vi "Host - Send Serial CMD (SubVI).vi"(5 "Access Restricted?":bool, 7 "Values":dbl[](array[numeric]), 10 "Camera Controls":T3, 11 "Data Cluster":T4={"VI References"=[], "Addresses"=[], "Pilot"=FALSE, "DO Data"=[], "Access Restricted?"=FALSE, "Pilot Control References"=[], "CoPilot Control References"=[], "cRIO Config"=[], "datalog Q"=refnum, "PS_P"={"AI"=[], "DI"=[], "DO"=[], "Serial"=[], "CPU"={"Total Load"=[], "Interrupt Load"=[], "Total Physical"=0.0, "Free Physical"=0.0, "Primary Disk Capacity"=0.0, "Primary Disk Free"=0.0}, "Stop"=FALSE, "DO Channel"=[]}, "PS_S"={"AI"=[], "DI"=[], "DO"=[], "Serial"=[], "CPU"={"Total Load"=[], "Interrupt Load"=[], "Total Physical"=0.0, "Free Physical"=0.0, "Primary Disk Capacity"=0.0, "Primary Disk Free"=0.0}, "Stop"=FALSE, "DO Channel"=[]}, "IDE_P"={"AI"=[], "DI"=[], "DO"=[], "Serial"=[], "CPU"={"Total Load"=[], "Interrupt Load"=[], "Total Physical"=0.0, "Free Physical"=0.0, "Primary Disk Capacity"=0.0, "Primary Disk Free"=0.0}, "Stop"=FALSE, "DO Channel"=[]}, "IDE_S"={"AI"=[], "DI"=[], "DO"=[], "Serial"=[], "CPU"={"Total Load"=[], "Interrupt Load"=[], "Total Physical"=0.0, "Free Physical"=0.0, "Primary Disk Capacity"=0.0, "Primary Disk Free"=0.0}, "Stop"=FALSE, "DO Channel"=[]}, "PDE_P"={"AI"=[], "DI"=[], "DO"=[], "Serial"=[], "CPU"={"Total Load"=[], "Interrupt Load"=[], "Total Physical"=0.0, "Free Physical"=0.0, "Primary Disk Capacity"=0.0, "Primary Disk Free"=0.0}, "Stop"=FALSE, "DO Channel"=[]}, "PDE_S"={"AI"=[], "DI"=[], "DO"=[], "Serial"=[], "CPU"={"Total Load"=[], "Interrupt Load"=[], "Total Physical"=0.0, "Free Physical"=0.0, "Primary Disk Capacity"=0.0, "Primary Disk Free"=0.0}, "Stop"=FALSE, "DO Channel"=[]}, "GUI References"={"Control Names"=[], "Control References"=[]}, "GUI Data"=[], "TCP - Serial"=[], "TCP-Serial Q"=refnum, "TCP Serial Ref"=[], "Data Sets"=[], "Last Data"=[], "Alarm Data"=[], "DI Data"=[], "Ack Data"=[], "Buzzer Data"=[], "Pilot DO"=[], "Co-Pilot DO"=[], "System Down?"=FALSE, "Log Data"=[], "Update Array"=[], "MCC Data Log"=[], "MCC Data Not"=refnum, "Thruster control"=[refnum, refnum, refnum, refnum, refnum, refnum, refnum, refnum, refnum], "waga notifier out"=refnum, "Wago  log"=[], "Thruster Cont"=[0.0, 0.0, 0.0, 0.0, 0.0, 0.0, 0.0, 0.0, 0.0], "Cam Cont"=[FALSE, FALSE, FALSE, FALSE, FALSE, TRUE], "PDE_P TH Cont"={"COM 10"=0.0, "COM 11"=0.0, "COM 12"=0.0, "COM 13"=0.0}, "PDE_S TH Cont"={"COM 10"=0.0, "COM 11"=0.0, "COM 12"=0.0, "COM 13"=0.0}} {"cRIO Config"."AI"."Interface Data"."Timing"."sample mode" items=["Finite Samples"=10178, "Continuous Samples"=10123, "Hardware Timed Single Point"=12522]; "cRIO Config"."Async"."Interface Data"."Data"."Minor Frame Count" min=5 max=8 step=1}) -> (2 "# elements in queue":i32)   [LabVIEW 2021]
uses:
  Controls/Host - GUI Data Cluster.ctl
  Analog Output/Controls/AO JSON Data Cluster.ctl
  Analog Output/Controls/AO Interface Data Cluster.ctl
  Analog Output/Controls/AO Channel Configuration Cluster.ctl
  Analog Output/Controls/AO Timing Cluster.ctl
  Digital Output/Controls/DIO Configuration cluster.ctl
  Digital Output/Controls/DIO Interface Data.ctl
  Digital Output/SubVIs/Digital Dynamic Cluster.ctl
  Async JSON Cluster.ctl
  Async Interface Data Cluster.ctl
  Async Serial/Controls/Async Serial Configuration Cluster.ctl
  Async Serial/Controls/Async Frame Info Cluster.ctl
  Async Serial/Controls/Async Message Info Cluster.ctl
  Controls/Host Data Cluster.ctl
  Main Engine/Controls/Main Engine CPU Info.ctl
  <userlib>/_OpenG.lib/comparison/comparison.llb/1D DBL Array Changed__ogtk.vi
  Controls/Global Variable.vi
  <userlib>/_OpenG.lib/comparison/comparison.llb/openg_comparison__ogtk.lvlib
panel:
  out "Changed":bool
  in  "Frame Info 2":T1[](array[typedef])=[{"Frame ID"=1, "Message Info"=[{"Message"=[16, 1, 111, 65, 32, 32, 0, 0, 16, 3, 20, 16, 1, 111, 65, 32, 32, 0, 0, 16, 3, 5], "Message Name"="cmd"}]}, {"Frame ID"=1, "Message Info"=[{"Message"=[16, 1, 111, 65, 32, 32, 0, 0, 16, 3, 20, 16, 1, 111, 65, 32, 32, 0, 0, 16, 3, 5], "Message Name"="cmd"}]}, {"Frame ID"=1, "Message Info"=[{"Message"=[16, 1, 111, 65, 32, 32, 0, 0, 16, 3, 20, 16, 1, 111, 65, 32, 32, 0, 0, 16, 3, 5], "Message Name"="cmd"}]}, {"Frame ID"=1, "Message Info"=[{"Message"=[16, 1, 111, 65, 32, 32, 0, 0, 16, 3, 20, 16, 1, 111, 65, 32, 32, 0, 0, 16, 3, 5], "Message Name"="cmd"}]}, {"Frame ID"=1, "Message Info"=[{"Message"=[16, 1, 111, 65, 32, 32, 0, 0, 16, 3, 20, 16, 1, 111, 65, 32, 32, 0, 0, 16, 3, 5], "Message Name"="cmd"}]}, {"Frame ID"=1, "Message Info"=[{"Message"=[16, 1, 111, 65, 32, 32, 0, 0, 16, 3, 20, 16, 1, 111, 65, 32, 32, 0, 0, 16, 3, 5], "Message Name"="cmd"}]}, {"Frame ID"=1, "Message Info"=[{"Message"=[16, 1, 111, 65, 32, 32, 0, 0, 16, 3, 20, 16, 1, 111, 65, 32, 32, 0, 0, 16, 3, 5], "Message Name"="cmd"}]}, {"Frame ID"=1, "Message Info"=[{"Message"=[16, 1, 111, 65, 32, 32, 0, 0, 16, 3, 20, 16, 1, 111, 65, 32, 32, 0, 0, 16, 3, 5], "Message Name"="cmd"}]}, {"Frame ID"=1, "Message Info"=[{"Message"=[111, 0, 0, 1], "Message Name"="LED"}]}, {"Frame ID"=1, "Message Info"=[{"Message"=[111, 0, 0, 1], "Message Name"="LED"}]}, {"Frame ID"=1, "Message Info"=[{"Message"=[111, 0, 0, 1], "Message Name"="LED"}]}, {"Frame ID"=0, "Message Info"=[{"Message"=[81, 1, 4, 7, 24, 255], "Message Name"="Camera cmd 1"}, {"Message"=[81, 1, 4, 7, 24, 255], "Message Name"="Camera cmd 2"}]}]
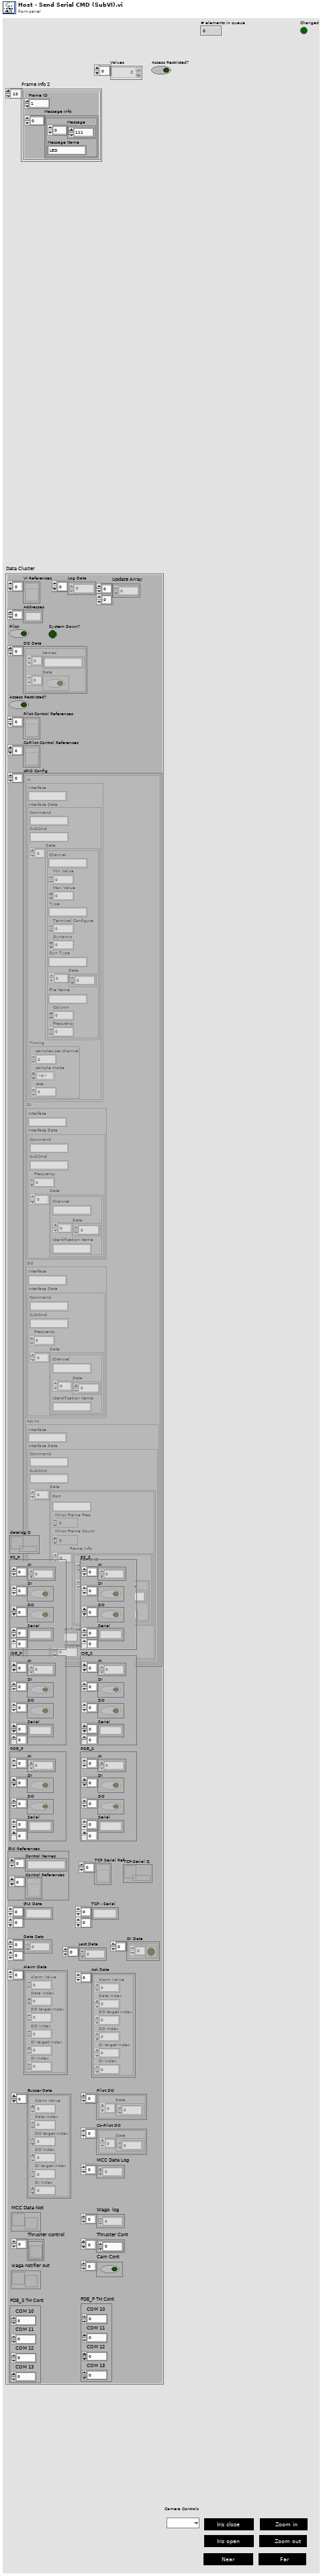
[diagram p1: front panel]
types:
  T1 = typedef "Async Frame Info Cluster.ctl" = cluster{"Frame ID":u16, "Message Info":T2[]}
  T2 = typedef "Async Message Info Cluster.ctl" = cluster{"Message":u8[], "Message Name":string}
  T3 = cluster{"Enum - Menu":enum16{"", "Camera 2", "Camera 1"}, "ZOOM IN":bool, "ZOOM OUT":bool, "IRIS OPEN":bool, "IRIS CLOSE":bool, "ZOOM OUT 2":bool, "IRIS CLOSE 2":bool}
  T4 = typedef "Host - GUI Data Cluster.ctl" = cluster{"VI References":refnum<vi>[], "Addresses":string[], "Pilot":bool, "DO Data":cluster{"Names":string[], "Data":bool[]}[], "Access Restricted?":bool, "Pilot Control References":refnum<vi>[], "CoPilot Control References":refnum<vi>[], "cRIO Config":cluster{"AI":T5, "DI":T9, "DO":T9, "Async":T12}[], "datalog Q":refnum<queue>, "PS_P":T15, "PS_S":T15, "IDE_P":T15, "IDE_S":T15, "PDE_P":T15, "PDE_S":T15, "GUI References":cluster{"Control Names":string[], "Control References":refnum<vi>[]}, "GUI Data":string[][], "TCP - Serial":string[][], "TCP-Serial Q":refnum<queue>, "TCP Serial Ref":refnum<vi>[], "Data Sets":dbl[][], "Last Data":dbl[], "Alarm Data":cluster{"Alarm Value":dbl, "Data Index":i32, "DO target Index":i32, "DO Index":i32, "DI target Index":i32, "DI Index":i32}[], "DI Data":cluster{bool[]}[], "Ack Data":cluster{"Alarm Value":dbl, "Data Index":i32, "DO target Index":i32, "DO Index":i32, "DI target Index":i32, "DI Index":i32}[], "Buzzer Data":cluster{"Alarm Value":dbl, "Data Index":i32, "DO target Index":i32, "DO Index":i32, "DI target Index":i32, "DI Index":i32}[], "Pilot DO":cluster{"Data":i32[]}[], "Co-Pilot DO":cluster{"Data":i32[]}[], "System Down?":bool, "Log Data":dbl[], "Update Array":i32[][], "MCC Data Log":dbl[], "MCC Data Not":refnum<notifier>, "Thruster control":refnum<vi>[], "waga notifier out":refnum<notifier>, "Wago  log":sgl[], "Thruster Cont":dbl[], "Cam Cont":bool[], "PDE_P TH Cont":cluster{"COM 10":dbl, "COM 11":dbl, "COM 12":dbl, "COM 13":dbl}, "PDE_S TH Cont":cluster{"COM 10":dbl, "COM 11":dbl, "COM 12":dbl, "COM 13":dbl}}
  T5 = typedef "AO JSON Data Cluster.ctl" = cluster{"Interface":string, "Interface Data":T6}
  T6 = typedef "AO Interface Data Cluster.ctl" = cluster{"Command":string, "SubCmd":string, "Data":T7[], "Timing":T8}
  T7 = typedef "AO Channel Configuration Cluster.ctl" = cluster{"Channel":string, "Min Value":dbl, "Max Value":dbl, "Type":string, "Terminal Configure":u16, "Dynamic":u8, "Dyn Type":string, "Data":dbl[], "File Name":string, "Column":i32, "Frequency":dbl}
  T8 = typedef "AO Timing Cluster.ctl" = cluster{"samples per channel":i32, "sample mode":i32, "rate":dbl}
  T9 = typedef "DIO Configuration cluster.ctl" = cluster{"Interface":string, "Interface Data":T10}
  T10 = typedef "DIO Interface Data.ctl" = cluster{"Command":string, "SubCmd":string, "Frequency":u16, "Data":T11[]}
  T11 = typedef "Digital Dynamic Cluster.ctl" = cluster{"Channel":string, "Data":u8[], "Identification Name":string}
  T12 = typedef "Async JSON Cluster.ctl" = cluster{"Interface":string, "Interface Data":T13}
  T13 = typedef "Async Interface Data Cluster.ctl" = cluster{"Command":string, "SubCmd":string, "Data":T14[]}
  T14 = typedef "Async Serial Configuration Cluster.ctl" = cluster{"Port":string, "Minor Frame Freq":u16, "Minor Frame Count":u16, "Frame Info":T1[], "Sensor Type":u16, "OIM Address":u16}
  T15 = typedef "Host Data Cluster.ctl" = cluster{"AI":dbl[], "DI":bool[], "DO":bool[], "Serial":string[][], "CPU":T16, "Stop":bool, "DO Channel":string[]}
  T16 = typedef "Main Engine CPU Info.ctl" = cluster{"Total Load":u32[], "Interrupt Load":u32[], "Total Physical":dbl, "Free Physical":dbl, "Primary Disk Capacity":dbl, "Primary Disk Free":dbl}
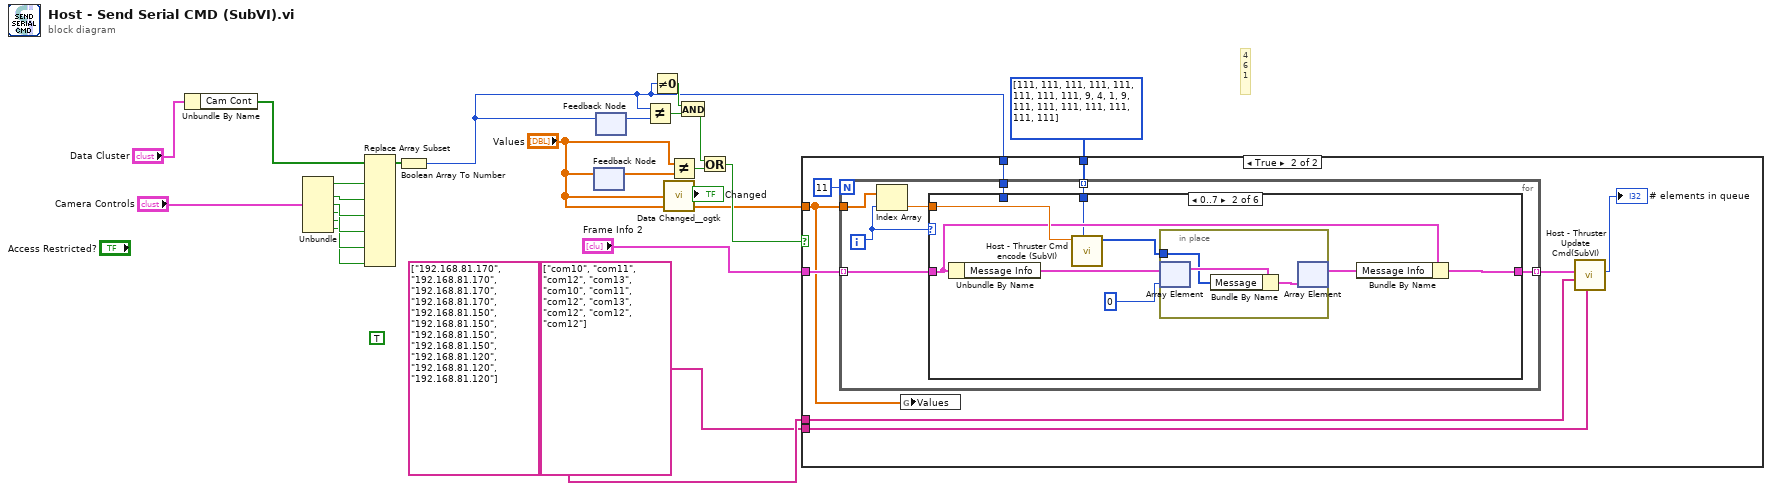
[diagram p0: block diagram]
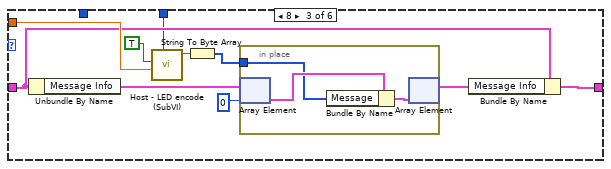
[diagram p4: hidden frame]
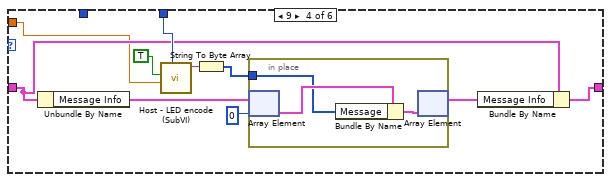
[diagram p5: hidden frame]
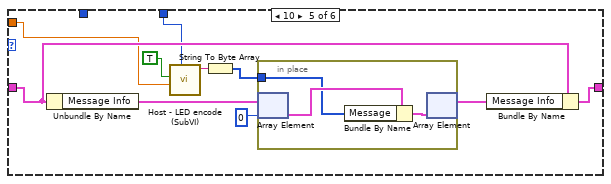
[diagram p6: hidden frame]
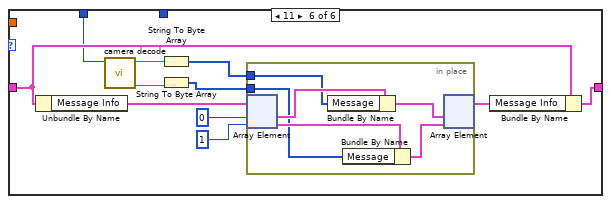
[diagram p7: hidden frame]
diagram:
  (unwired) TRUE
  # "4\n6\n1"
  n1 = Unbundle By Name("Data Cluster") -> ("Cam Cont"=w5:bool[])
  n2 = Unbundle("Camera Controls") -> ("ZOOM IN"=w13:bool, "ZOOM OUT"=w12:bool, "IRIS OPEN"=w11:bool, "IRIS CLOSE"=w10:bool, "ZOOM OUT 2"=w9:bool, "IRIS CLOSE 2"=w8:bool)  [unwired: 1 out]
  n3 = Replace Array Subset(array=w5, new element #1=w13, new element #2=w12, new element #3=w11, new element #4=w10, new element #5=w9, new element #6=w8) -> (w7:bool[])  [unwired: 6 in]
  n4 = Boolean Array To Number(Boolean array=w7) -> (number=w4:u32)
  n5 = feedback #1() -> (w19:dbl[])  [unwired: 1 in]
  n6 = feedback-in #1("Values") -> ()
  n7 = feedback #2() -> (w18:u32)  [unwired: 1 in]
  n8 = feedback-in #2(w4) -> ()
  n9 = Not Equal?(x=w4, y=w18) -> (x != y?=w17:bool)
  n10 = Not Equal To 0?(x=w4) -> (x != 0?=w15:bool)
  n11 = call-poly <userlib>:"Data Changed__ogtk.vi"("1D DBL Array"="Values") -> ("Changed"=→"Changed":bool)
  n12 = Not Equal?(x="Values", y=w19) -> (x != y?=w24:bool)
  n13 = And(x=w15, y=w17) -> (x .and. y?=w16:bool)
  n14 = Or(x=w16, y=w24) -> (x .or. y?=w3:bool)
  n15 = case shown="True" w3 {
    tunnel: "Values" -> [_ w28]
    tunnel: "Frame Info 2" -> [_ w33]
    tunnel: string[] ["192.168.81.170", "192.168.81.170", "192.168.81.170", "192.168.81.170", "192.168.81.150", "192.168.81.150", "192.168.81.150", "192.168.81.150", "192.168.81.120", "192.168.81.120", "192.168.81.120"] ("IP Address") -> [_ w31]
    tunnel: string[] ["com10", "com11", "com12", "com13", "com10", "com11", "com12", "com13", "com12", "com12", "com12"] ("Com") -> [_ w30]
    tunnel: u16[] [111, 111, 111, 111, 111, 111, 111, 111, 9, 4, 1, 9, 111, 111, 111, 111, 111, 111, 111] -> [_ w29]
    tunnel: w4 -> [_ w27]
    frame False {
    }
    frame True {
      n16 = for {
        N: 11 -> [_]
        tunnel: w28 -> [w36]
        tunnel: w33 -> [w34] mode=indexing
        tunnel: [w40] -> w32 mode=indexing
        tunnel: w29 -> [w39] mode=indexing
        tunnel: w27 -> [w38]
        i -> [w35]
        n17 = Index Array(array=w36, index=w35) -> (element=w37:dbl)
        n18 = case shown="0..7" w35 {
          tunnel: w37 -> [_ w48 w61 w66 w79 _]
          tunnel: w34 -> [_ w47 w60 w67 w81 w97]
          tunnel: [_ w42 w56 w65 w80 w96] -> w40
          tunnel: w39 -> [_ w41 w54 w68 w78 _]
          tunnel: w38 -> [_ _ _ _ _ w95]
          frame Default {
          }
          frame 0..7 {
            n19 = Unbundle By Name(w47) -> ("Message Info"=w46:T2[])
            n20 = call "Host - Thruster Cmd encode (SubVI).vi"("Address"=w41, "Thruster ctrl"=w48) -> ("cmd Array"=w44:u32[])  [unwired: 9 in]
            n21 = in-place {
              in-place-border: w44 -> [w50]
              n22 = in-place-array #3(w46, 0) -> (w51:T2)
              n23 = Bundle By Name(cluster=w51, "Message"=w50) -> (w49:T2)
              n24 = in-place-array #3(w49) -> (w43:T2[])  [unwired: 1 out]
            }
            n25 = Bundle By Name(cluster=w47, "Message Info"=w43) -> (w42:T1)
          }
          frame 8 {
            n26 = Unbundle By Name(w60) -> ("Message Info"=w59:T2[])
            n27 = call "Host - LED encode (SubVI).vi"("Address"=w54, "Dim Ctrl"=w61, "led"=TRUE) -> ("Command"=w52:string)  [unwired: 7 in, 1 out]
            n28 = String To Byte Array(string=w52) -> (unsigned byte array=w55:u8[])
            n29 = in-place {
              in-place-border: w55 -> [w63]
              n30 = in-place-array #4(w59, 0) -> (w64:T2)
              n31 = Bundle By Name(cluster=w64, "Message"=w63) -> (w62:T2)
              n32 = in-place-array #4(w62) -> (w57:T2[])  [unwired: 1 out]
            }
            n33 = Bundle By Name(cluster=w60, "Message Info"=w57) -> (w56:T1)
          }
          frame 9 {
            n34 = Unbundle By Name(w67) -> ("Message Info"=w74:T2[])
            n35 = call "Host - LED encode (SubVI).vi"("Address"=w68, "Dim Ctrl"=w66, "led"=TRUE) -> ("Command"=w69:string)  [unwired: 7 in, 1 out]
            n36 = String To Byte Array(string=w69) -> (unsigned byte array=w71:u8[])
            n37 = in-place {
              in-place-border: w71 -> [w76]
              n38 = in-place-array #5(w74, 0) -> (w77:T2)
              n39 = Bundle By Name(cluster=w77, "Message"=w76) -> (w75:T2)
              n40 = in-place-array #5(w75) -> (w72:T2[])  [unwired: 1 out]
            }
            n41 = Bundle By Name(cluster=w67, "Message Info"=w72) -> (w65:T1)
          }
          frame 10 {
            n42 = Unbundle By Name(w81) -> ("Message Info"=w87:T2[])
            n43 = call "Host - LED encode (SubVI).vi"("Address"=w78, "Dim Ctrl"=w79, "led"=TRUE) -> ("Command"=w82:string)  [unwired: 7 in, 1 out]
            n44 = String To Byte Array(string=w82) -> (unsigned byte array=w84:u8[])
            n45 = in-place {
              in-place-border: w84 -> [w89]
              n46 = in-place-array #6(w87, 0) -> (w90:T2)
              n47 = Bundle By Name(cluster=w90, "Message"=w89) -> (w88:T2)
              n48 = in-place-array #6(w88) -> (w85:T2[])  [unwired: 1 out]
            }
            n49 = Bundle By Name(cluster=w81, "Message Info"=w85) -> (w80:T1)
          }
          frame 11 {
            n50 = Unbundle By Name(w97) -> ("Message Info"=w101:T2[])
            n51 = call "camera decode.vi"("Numeric"=w95) -> ("command 2"=w92:string, "command 1"=w94:string)  [unwired: 9 in]
            n52 = String To Byte Array(string=w94) -> (unsigned byte array=w98:u8[])
            n53 = String To Byte Array(string=w92) -> (unsigned byte array=w91:u8[])
            n54 = in-place {
              in-place-border: w98 -> [w106]
              in-place-border: w91 -> [w103]
              n55 = in-place-array #7(w101, 0, 1) -> (w107:T2, w104:T2)
              n56 = Bundle By Name(cluster=w107, "Message"=w106) -> (w105:T2)
              n57 = Bundle By Name(cluster=w104, "Message"=w103) -> (w102:T2)
              n58 = in-place-array #7(w105, w102) -> (w99:T2[])  [unwired: 2 out]
            }
            n59 = Bundle By Name(cluster=w97, "Message Info"=w99) -> (w96:T1)
          }
        }
      }
      n60 = global write "Global Variable.vi" "Values"(w28) -> ()
      n61 = call "Host - Thruster Update Cmd(SubVI).vi"("Com"=w30, "IP Address"=w31, "Serial Input"=w32) -> ("# elements in queue"=→"# elements in queue":i32)  [unwired: 7 in, 1 out]
    }
  }
